vi "Area and time calculation(SubVI).vi"(3 "Array in 2":dbl[](array[numeric]), 4 "Array in":dbl[](array[numeric])) -> (1 "Array out":dbl[][](array[numeric]))   [LabVIEW 2014]
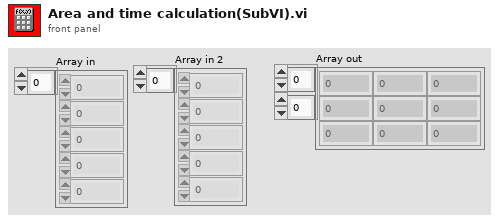
[diagram p1: front panel]
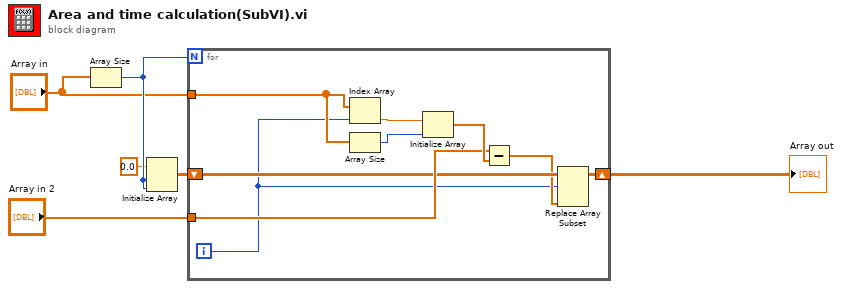
[diagram p0: block diagram]
diagram:
  n1 = Array Size(array="Array in") -> (size(s)=w5:i32)
  n2 = Initialize Array(0.0 ("element"), w5, w5) -> (w3:dbl[][])
  n3 = for {
    N: w5 -> [_]
    tunnel: "Array in" -> [w14]
    tunnel: "Array in 2" -> [w12]
    shift-right: [w7] -> w6
    shift-left: w3 -> [w10]
    i -> [w8]
    n4 = Index Array(array=w14, index=w8) -> (element=w15:dbl)
    n5 = Array Size(array=w14) -> (size(s)=w11:i32)
    n6 = Initialize Array(w15, w11) -> (w13:dbl[])
    n7 = Subtract(x=w12, y=w13) -> (x-y=w9:dbl[])
    n8 = Replace Array Subset(array=w10, new element=w9, index (row)=w8) -> (w7:dbl[][])  [unwired: 1 in]
  }
  "Array out" <- w6
